vi "Get SMO Name.vi"(8 "error in (no error)":errorcluster, 11 "Instrument.Transport in":refnum<class "Inst.Transport.lvclass">) -> (0 "error out":errorcluster, 2 "SMO Name":string, 3 "Instrument.Transport out":refnum<class "Inst.Transport.lvclass">)   [LabVIEW 2019, in "Inst.Transport.lvclass"]
uses:
  Inst.Transport.lvclass
  <userlib>/LevyLab/Instrument Framework/Instrument Types/SCPI/Instrument.SCPI.lvclass
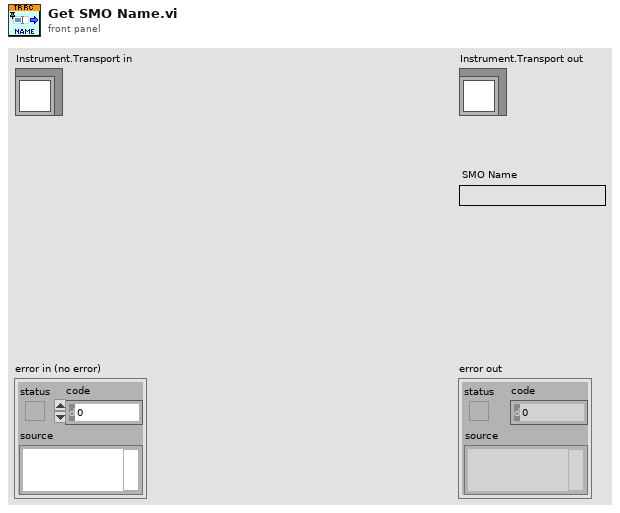
[diagram p1: front panel]
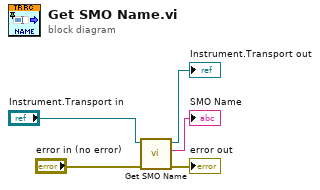
[diagram p0: block diagram]
diagram:
  n1 = call-parent "Get SMO Name.vi"("error in (no error)"="error in (no error)", "Instrument in"="Instrument.Transport in") -> ("error out"=→"error out":errorcluster, "SMO Name"=→"SMO Name":string, "Instrument out"=→"Instrument.Transport out":refnum<class "Inst.Transport.lvclass">)  [unwired: 7 in]
